vi "MessageName.vi"() -> (2 "MessageName":string)   [LabVIEW 2020, in "Double.lvlib"]
uses:
  Double.lvlib
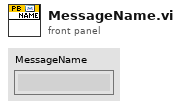
[diagram p1: front panel]
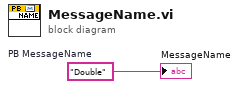
[diagram p0: block diagram]
diagram:
  w1 = "Double"  # PB MessageName
  "MessageName" <- w1
